vi "PM100D_Fetch.vi"(0 "VISA In":refnum<visa-resource-name>, 1 "Timeout":i32, 2 "error in":errorcluster) -> (3 "VISA Out":refnum<visa-resource-name>, 4 "ReadValue":string, 5 "Boolean":bool, 6 "error out":errorcluster)   [LabVIEW 2011]
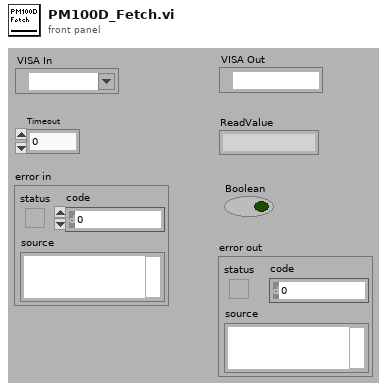
[diagram p1: front panel]
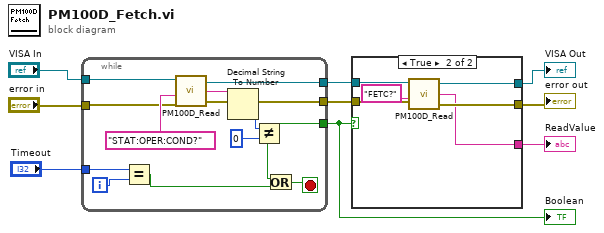
[diagram p0: block diagram]
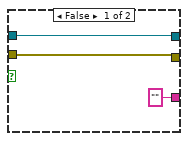
[diagram p2: hidden frame]
diagram:
  n1 = while {
    tunnel: "VISA In" -> [w18]
    tunnel: [w17] -> w3
    tunnel: [w13] -> w8
    tunnel: "error in" -> [w12]
    tunnel: [w11] -> w2
    tunnel: "Timeout" -> [w10]
    i -> [w16]
    stop <- w15 stop-if-true
    n2 = Equal?(x=w10, y=w16) -> (x = y?=w14:bool)
    n3 = call "PM100D_Read.vi"("error in (no error)"=w12, "Command"="STAT:OPER:COND?", "VISA in"=w18) -> ("error out"=w11:errorcluster, "ReadValue"=w21:string, "VISA out"=w17:refnum<visa-resource-name>)  [unwired: 1 in]
    n4 = Decimal String To Number(string=w21) -> (number=w20:i32)  [unwired: 2 in, 1 out]
    n5 = Not Equal?(x=w20, y=0) -> (x != y?=w13:bool)
    n6 = Or(x=w13, y=w14) -> (x .or. y?=w15:bool)
  }
  "Boolean" <- w8
  n7 = case shown="True" w8 {
    tunnel: w3 -> [w25 w30]
    tunnel: [w25 w29] -> w6
    tunnel: w2 -> [w24 w28]
    tunnel: [w24 w27] -> w7
    tunnel: ["" ("ReadValue") w26] -> w9
    frame False {
    }
    frame True {
      n8 = call "PM100D_Read.vi"("error in (no error)"=w28, "Command"="FETC?", "VISA in"=w30) -> ("error out"=w27:errorcluster, "ReadValue"=w26:string, "VISA out"=w29:refnum<visa-resource-name>)  [unwired: 1 in]
    }
  }
  "ReadValue" <- w9
  "error out" <- w7
  "VISA Out" <- w6
